vi "comport 2.vi"(9 "x":u8=100, 10 "error in (no error)":errorcluster, 11 "VISA resource name":refnum<visa-resource-name>) -> (1 "error out":errorcluster, 2 "Numeric":u8, 3 "VISA resource name out":refnum<visa-resource-name>)   [LabVIEW 2020]
uses:
  <vilib>/Instr/_visa.llb/VISA Configure Serial Port (Instr).vi
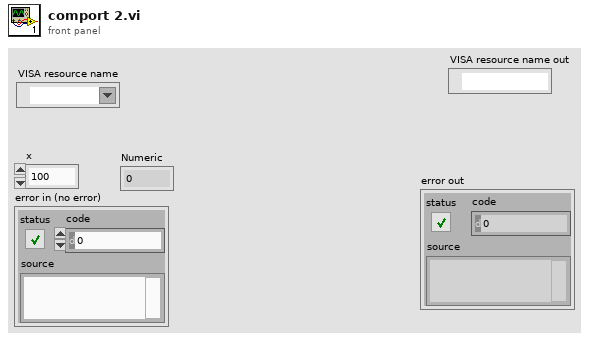
[diagram p1: front panel]
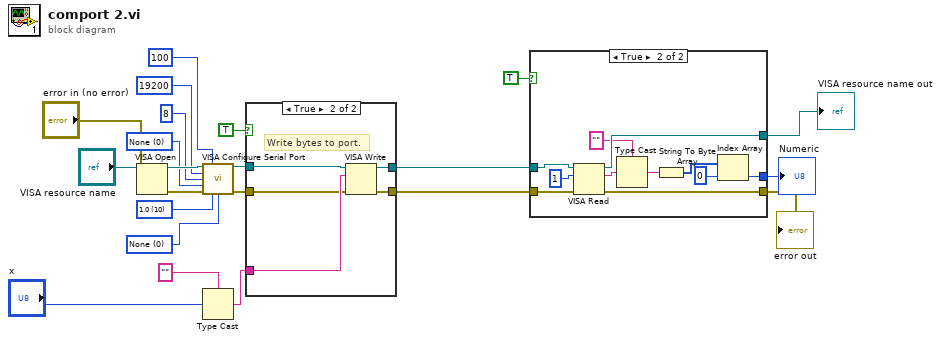
[diagram p0: block diagram]
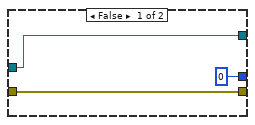
[diagram p3: hidden frame]
diagram:
  w9 = u16 0 items=["None"=0, "XON/XOFF"=1, "RTS/CTS"=2, "DTR/DSR"=4] ("flow control")
  w8 = u16 10 items=["1.0"=10, "1.5"=15, "2.0"=20] ("stop bits")
  w7 = u16 0 items=["None", "Odd", "Even", "Mark", "Space"] ("parity")
  n1 = VISA Open(error in (no error)="error in (no error)", VISA resource name="VISA resource name") -> (VISA resource name=w20:refnum<visa-resource-name>, error out=w21:errorcluster)  [unwired: 3 in]
  n2 = call-poly "VISA Configure Serial Port"("VISA resource name"=w20, "timeout (10sec)"=u32 100, "baud rate (9600)"=u32 19200 ("baud rate"), "data bits (8)"=u16 8 ("data bits"), "parity (0:none)"=w7, "error in (no error)"=w21, "stop bits (10: 1 bit)"=w8, "flow control (0:none)"=w9) -> ("VISA resource name out"=w6:refnum<visa-resource-name>, "error out"=w5:errorcluster)  [unwired: 1 in, 5 out]
  n3 = Type Cast(type="", x="x") -> (*(type *) &x=w13:string)
  n4 = case shown="True" TRUE {
    tunnel: [w24 w29] -> w11
    tunnel: w6 -> [w23 w26]
    tunnel: w5 -> [w24 w25]
    tunnel: [w23 w28] -> w12
    tunnel: w13 -> [_ w27]
    frame False {
    }
    frame True {
      # "Write bytes to port."
      n5 = VISA Write(VISA resource name=w26, write buffer=w27, error in (no error)=w25) -> (VISA resource name out=w28:refnum<visa-resource-name>, error out=w29:errorcluster)  [unwired: 1 out]
    }
  }
  n6 = case shown="True" TRUE {
    tunnel: w11 -> [w32 w40]
    tunnel: [w32 w43] -> w1
    tunnel: [w31 w42] -> w3
    tunnel: w12 -> [w31 w41]
    tunnel: [u8 0 w33] -> w19
    frame False {
    }
    frame True {
      n7 = VISA Read(VISA resource name=w41, byte count=u32 1, error in (no error)=w40) -> (VISA resource name out=w42:refnum<visa-resource-name>, read buffer=w38:string, error out=w43:errorcluster)  [unwired: 1 out]
      n8 = Type Cast(type="", x=w38) -> (*(type *) &x=w36:string)
      n9 = String To Byte Array(string=w36) -> (unsigned byte array=w35:u8[])
      n10 = Index Array(array=w35, index=0) -> (element=w33:u8)
    }
  }
  "Numeric" <- w19
  "VISA resource name out" <- w3
  "error out" <- w1
